vi "Send Update.vi"(8 "error in (no error)":errorcluster, 10 "Send Data":string, 11 "NodeRed-LV-Interface in":refnum<class "NodeRed-LV-Interface.lvclass">) -> (0 "error out":errorcluster, 3 "NodeRed-LV-Interface out":refnum<class "NodeRed-LV-Interface.lvclass">)   [LabVIEW 2020, in "NodeRed-LV-Interface.lvclass"]
uses:
  NodeRed-LV-Interface.lvclass
  NodeRed-LV-Interface.lvclass/NodeRed-LV-Interface.ctl
  Read Receive Data.vi
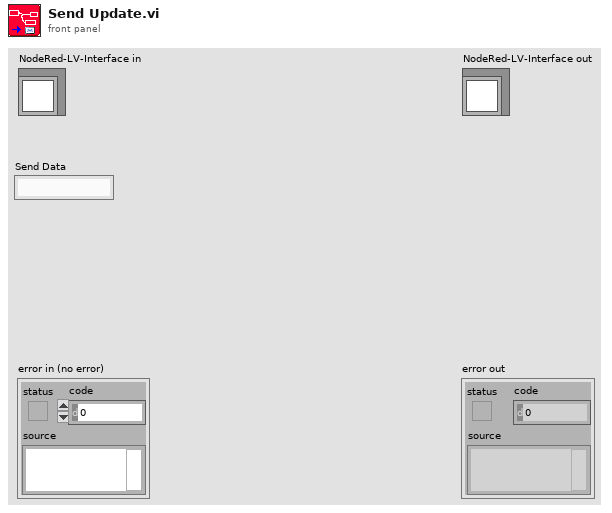
[diagram p1: front panel]
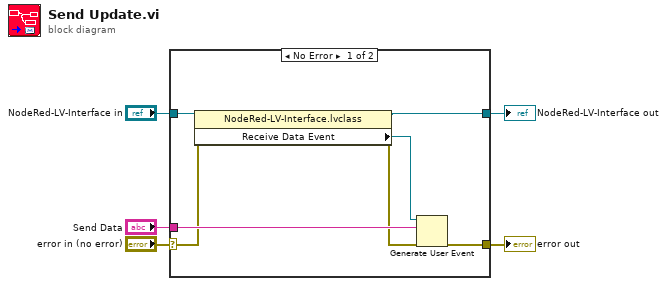
[diagram p0: block diagram]
diagram:
  n1 = case shown="No Error" "error in (no error)" {
    selector: "error in (no error)" -> [w7 w14]
    tunnel: [w8 w14] -> w4
    tunnel: [w11 w13] -> w3
    tunnel: "NodeRed-LV-Interface in" -> [w12 w13]
    tunnel: "Send Data" -> [w9 _]
    frame No Error {
      n2 = property class="NodeRed-LV-Interface.lvclass"(reference=w12, error in=w7) -> (reference out=w11:refnum<class "NodeRed-LV-Interface.lvclass">, error out=w6:errorcluster, "Receive Data Event"=w10:refnum<user-event>)
      n3 = Generate User Event(user event=w10, event data cluster=w9, error in=w6) -> (error out=w8:errorcluster)  [unwired: 1 in, 1 out]
    }
    frame Error {
    }
  }
  "error out" <- w4
  "NodeRed-LV-Interface out" <- w3
